vi "Generate signal on external trigger.vi"() -> ()   [LabVIEW 2010]
doc: "This example shows how to program Red Pitaya to generate analog signal on external trigger. Red Pitaya will first wait for trigger from external source and start generating desired signal right after trigger condition is meet. Red Pitaya is able to generate signals in range from DC to 50 MHz with output voltage range from -1 to 1 Volt. Generated signal can be observed by Red Pitaya Oscilloscope WEB application. To run it, just open web browser, input Red Pitaya IP and start Oscilloscope."
uses:
  RedPitaya.lvlib
panel:
  in  "Number of repeated Bursts":i32=1 min=-1 max=50000
  in  "Number of generated Signals / Burst":i32=1 min=-1 max=50000
  in  "Trigger Source":u16(ring)=1 items=["", "EXT_PE", "EXT_NE", "INT", "GATED", "IMM", "IMM BOTH"]
  in  "Total Time of One Burst":i32=-1
  in  "Waveform Function":u16(ring)=1 items=["", "Sine", "Square", "Triangle", "Sawtooth UP", "Sawtooth Down", "PWM"]
  in  "Channel (1|2)":u16(ring)=1 items=["Channel 1"=1, "Channel 2"=2]
  in  "Amplitude":dbl=1.0
  in  "Frequency":i32=200
  in  "IP address":string="192.168.1.100"
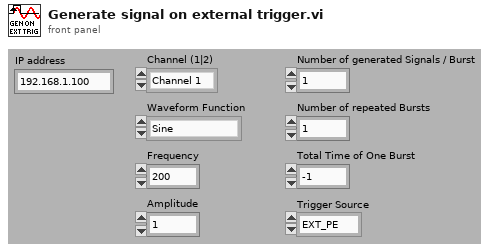
[diagram p1: front panel]
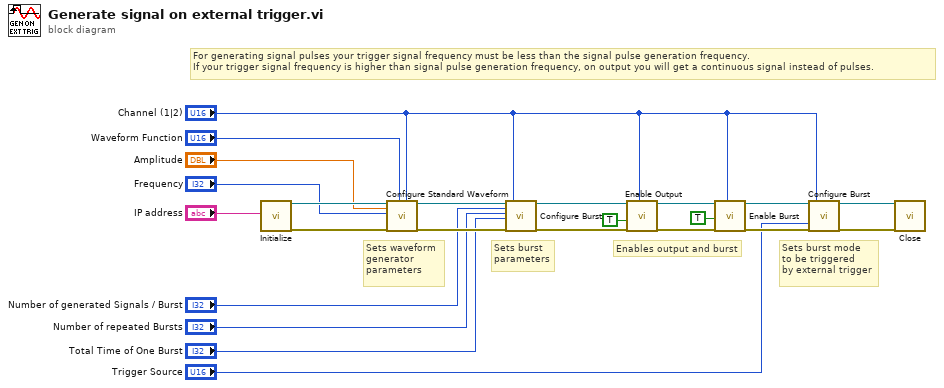
[diagram p0: block diagram]
diagram:
  # "For generating signal pulses your trigger signal frequency must be less than the signal pulse generation frequency.\nIf your trigger signal frequency is higher than signal pulse generation frequency, on output you will get a continuous signal instead of pulses."
  # "Sets burst mode\nto be triggered\nby external trigger"
  # "Enables output and burst"
  # "Sets burst\nparameters"
  # "Sets waveform\ngenerator\nparameters"
  n1 = call "Initialize.vi"("IP address"="IP address") -> ("RedPitaya connection out"=w21:refnum<k5>, "error out"=w20:errorcluster)  [unwired: 17 in]
  n2 = call "Configure Standard Waveform.vi"("RedPitaya connection in"=w21, "Amplitude (V)"="Amplitude", "Frequency"="Frequency", "error in"=w20, "Channel #"="Channel (1|2)", "Waveform Function"="Waveform Function") -> ("RedPitaya connection out"=w19:refnum<k5>, "error out"=w17:errorcluster)  [unwired: 12 in]
  n3 = call "Configure Burst.vi"("RedPitaya connection in"=w19, "Number of generated Signals / Burst"="Number of generated Signals / Burst", "Number of repeated Bursts"="Number of repeated Bursts", "Total time of One Burst"="Total Time of One Burst", "error in"=w17, "Channel #"="Channel (1|2)") -> ("RedPitaya connection out"=w18:refnum<k5>, "error out"=w16:errorcluster)  [unwired: 12 in]
  n4 = call "Enable Output.vi"("RedPitaya connection in"=w18, "Generation (T: Enable)"=TRUE, "error in"=w16, "Channel #"="Channel (1|2)") -> ("RedPitaya connection out"=w15:refnum<k5>, "error out"=w14:errorcluster)  [unwired: 14 in]
  n5 = call "Enable Burst.vi"("RedPitaya connection in"=w15, "Generation (T: Enable)"=TRUE, "error in"=w14, "Channel #"="Channel (1|2)") -> ("RedPitaya connection out"=w12:refnum<k5>, "error out"=w11:errorcluster)  [unwired: 14 in]
  n6 = call "Configure Burst.vi"("RedPitaya connection in"=w12, "Trigger Source"="Trigger Source", "error in"=w11, "Channel #"="Channel (1|2)") -> ("RedPitaya connection out"=w9:refnum<k5>, "error out"=w10:errorcluster)  [unwired: 14 in]
  n7 = call "Close.vi"("RedPitaya connection in"=w9, "error in"=w10) -> ()  [unwired: 17 in, 1 out]
